vi "CmdListGen.vi"() -> (0 "队列输出":refnum<queue>)   [LabVIEW 2012]
panel:
  in  "Msg":T1
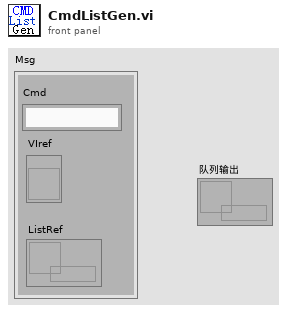
[diagram p1: front panel]
types:
  T1 = cluster{"Cmd":string, "VIref":refnum<vi>, "ListRef":refnum<queue>}
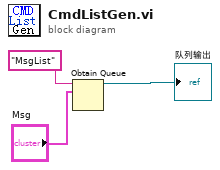
[diagram p0: block diagram]
diagram:
  n1 = Obtain Queue(name (unnamed)="MsgList" ("名称（未命名）"), element data type="Msg") -> (queue out=→"队列输出":refnum<queue>)  [unwired: 3 in, 2 out]
